vi "MagnitudesToPeaksFreqArray.vi"(2 "Size":i32=6, 3 "magnitude":cluster{"f0":dbl, "df":dbl, "magnitude":dbl[]}) -> (0 "# found":i32, 1 "Para Cubo":dbl[][](array[numeric]))   [LabVIEW 2016]
uses:
  <vilib>/measure/mamon.llb/Waveform Peak Detection for 1 Chan.vi
  <vilib>/measure/NI_MAPro.lvlib
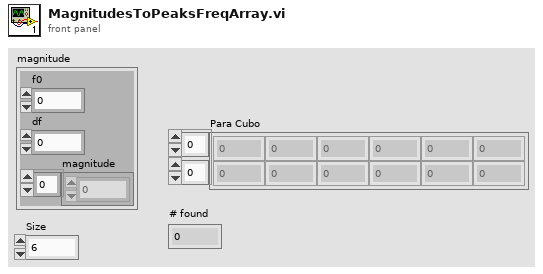
[diagram p1: front panel]
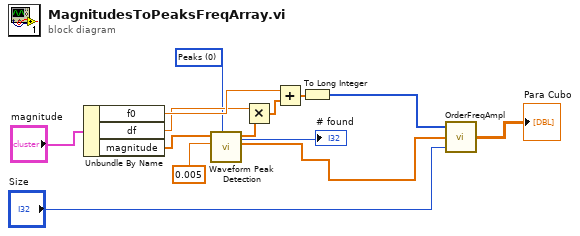
[diagram p0: block diagram]
diagram:
  w5 = u16 0 items=["Peaks", "Valleys"] ("peaks/valleys")
  n1 = Unbundle By Name("magnitude") -> ("f0"=w9:dbl, "df"=w7:dbl, "magnitude"=w4:dbl[])
  n2 = call-poly <vilib>:"Waveform Peak Detection.vi"("peaks/valleys"=w5, "threshold"=0.005, "Signal In"=w4) -> ("Amplitudes"=w12:dbl[], "Locations"=w6:dbl[], "# found"=→"# found":i32)  [unwired: 4 in, 2 out]
  n3 = Multiply(x=w7, y=w6) -> (x*y=w8:dbl[])
  n4 = Add(x=w9, y=w8) -> (x+y=w10:dbl[])
  n5 = To Long Integer(number=w10) -> (32bit integer=w11:i32[])
  n6 = call "OrderFreqAmpl.vi"("Size"="Size", "Amplitude"=w12, "Frequencies"=w11) -> ("appended array"=→"Para Cubo":dbl[][])
